vi "Trajectory Adaptation Algorithm_v4.vi"(0 "baseline (x,y,z)":dbl[](array[numeric])=[0.0, 5.0, 0.0] format="%.2f", 5 "assigned (x,y,z)":dbl[](array[numeric])=[0.0, 5.0, 0.0], 7 "Tt":dbl, 9 "Th":dbl, 11 "index":i32) -> (4 "rerouted (x,y,z)":dbl[](array[numeric])=[0.0, 5.0, 0.0])   [LabVIEW 2010]
doc: "This VI ramps linearly to an assigned point, interrupt is possible if index is reset to 0."
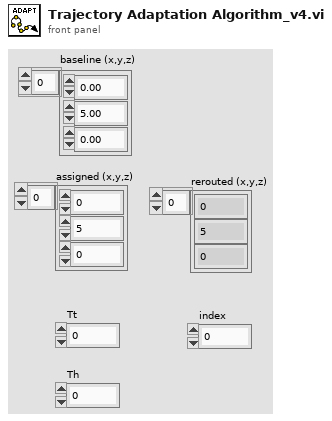
[diagram p1: front panel]
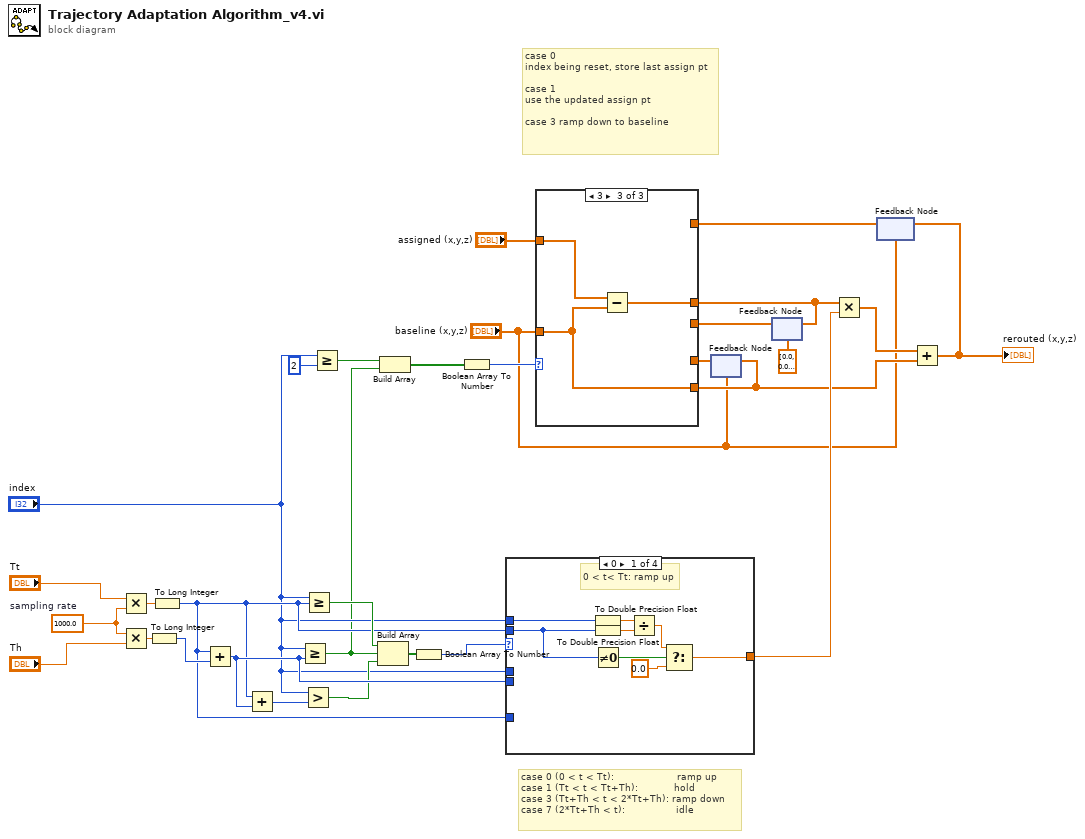
[diagram p0: block diagram]
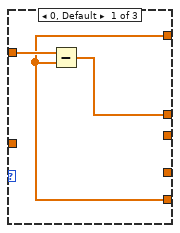
[diagram p2: hidden frame]
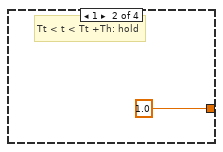
[diagram p4: hidden frame]
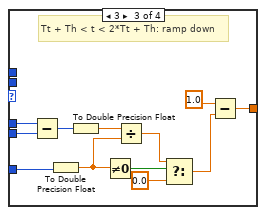
[diagram p5: hidden frame]
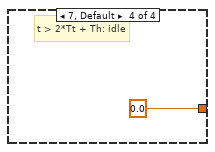
[diagram p6: hidden frame]
diagram:
  w27 = 1000.0  # sampling rate
  # "case 0 \nindex being reset, store last assign pt\n\ncase 1 \nuse the updated assign pt\n\ncase 3 ramp down to baseline"
  # "case 0 (0 < t < Tt):                     ramp up\ncase 1 (Tt < t < Tt+Th):            hold\ncase 3 (Tt+Th < t < 2*Tt+Th): ramp down\ncase 7 (2*Tt+Th < t):                 idle"
  n1 = Multiply(x="Tt", y=w27) -> (x*y=w29:dbl)
  n2 = Multiply(x=w27, y="Th") -> (x*y=w30:dbl)
  n3 = To Long Integer(number=w30) -> (32bit integer=w28:i32)
  n4 = To Long Integer(number=w29) -> (32bit integer=w20:i32)
  n5 = Add(x=w20, y=w28) -> (x+y=w21:i32)
  n6 = Add(x=w20, y=w21) -> (x+y=w24:i32)
  n7 = Greater Or Equal?(x="index", y=w21) -> (x >= y?=w9:bool)
  n8 = Greater?(x="index", y=w24) -> (0:w12:bool)
  n9 = Greater Or Equal?(x="index", y=w20) -> (x >= y?=w26:bool)
  n10 = Greater Or Equal?(x="index", y=2) -> (x >= y?=w16:bool)
  n11 = Build Array(w26, w9, w12) -> (w25:bool[])
  n12 = Build Array(w16, w9) -> (w18:bool[])
  n13 = Boolean Array To Number(Boolean array=w25) -> (number=w10:u32)
  n14 = Boolean Array To Number(Boolean array=w18) -> (number=w17:u32)
  n15 = case shown="0" w10 {
    tunnel: w20 -> [w35 _ _ _]
    tunnel: "index" -> [w36 _ _ _]
    tunnel: [w32 1.0 w48 0.0] -> w14
    tunnel: "index" -> [_ _ w50 _]
    tunnel: w21 -> [_ _ w49 _]
    tunnel: w20 -> [_ _ w45 _]
    frame 0 {
      # "0 < t< Tt: ramp up"
      n16 = To Double Precision Float(number=w36) -> (double precision float=w38:dbl)
      n17 = To Double Precision Float(number=w35) -> (double precision float=w37:dbl)
      n18 = Not Equal To 0?(x=w35) -> (x != 0?=w34:bool)
      n19 = Divide(x=w38, y=w37) -> (x/y=w33:dbl)
      n20 = Select(t=w33, s=w34, f=0.0) -> (s? t:f=w32:dbl)
    }
    frame 1 {
      # "Tt < t < Tt +Th: hold"
    }
    frame 3 {
      # "Tt + Th < t < 2*Tt + Th: ramp down"
      n21 = Subtract(x=w50, y=w49) -> (x-y=w47:i32)
      n22 = To Double Precision Float(number=w45) -> (double precision float=w42:dbl)
      n23 = To Double Precision Float(number=w47) -> (double precision float=w46:dbl)
      n24 = Not Equal To 0?(x=w42) -> (x != 0?=w44:bool)
      n25 = Divide(x=w46, y=w42) -> (x/y=w40:dbl)
      n26 = Select(t=w40, s=w44, f=0.0) -> (s? t:f=w41:dbl)
      n27 = Subtract(x=1.0, y=w41) -> (x-y=w48:dbl)
    }
    frame 7, Default {
      # "t > 2*Tt + Th: idle"
    }
  }
  n28 = feedback #1("baseline (x,y,z)") -> (w5:dbl[])
  n29 = feedback #2(dbl[] [0.0, 0.0, 0.0]) -> (w7:dbl[])
  n30 = feedback #3("baseline (x,y,z)") -> (w3:dbl[])
  n31 = case shown="3" w17 {
    tunnel: w3 -> [w53 _ _]
    tunnel: "assigned (x,y,z)" -> [w55 _ w60]
    tunnel: "baseline (x,y,z)" -> [_ _ w58]
    tunnel: [w54 w57 w59] -> w8
    tunnel: [w53 w56 w58] -> w2
    tunnel: w7 -> [_ w57 _]
    tunnel: w5 -> [_ w56 _]
    frame 0, Default {
      n32 = Subtract(x=w55, y=w53) -> (x-y=w54:dbl[])
    }
    frame 1 {
    }
    frame 3 {
      n33 = Subtract(x=w60, y=w58) -> (x-y=w59:dbl[])
    }
  }
  n34 = feedback-in #1(w2) -> ()
  n35 = feedback-in #2(w8) -> ()
  n36 = Multiply(x=w8, y=w14) -> (x*y=w13:dbl[])
  n37 = Add(x=w13, y=w2) -> (x+y=w4:dbl[])
  "rerouted (x,y,z)" <- w4
  n38 = feedback-in #3(w4) -> ()
